vi "Close.vi"(8 "error in (no error)":errorcluster, 11 "Digital Output in":refnum<class "Digital Output.lvclass">) -> (0 "error out":errorcluster)   [LabVIEW 2021, in "Digital Output.lvlib" / "Digital Output.lvclass"]
uses:
  Digital Output.lvclass
  Digital Output.lvclass/Digital Output.ctl
  <vilib>/DAQmx/write.llb/DAQmx Write (Digital Bool 1Line 1Point).vi
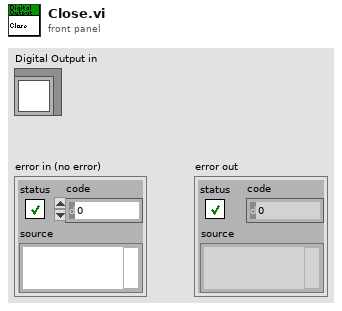
[diagram p1: front panel]
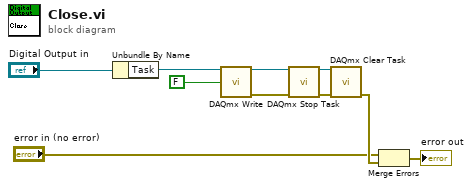
[diagram p0: block diagram]
diagram:
  n1 = Unbundle By Name("Digital Output in") -> ("Task"=w6:refnum<k21>)
  n2 = call-poly <vilib>:"DAQmx Write.vi"("task/channels in"=w6, "data"=FALSE) -> ("task out"=w5:refnum<k21>, "error out"=w7:errorcluster)  [unwired: 11 in, 1 out]
  n3 = call <vilib>:"DAQmx Stop Task.vi"("task/channels in"=w5, "error in"=w7) -> ("task out"=w10:refnum<k21>, "error out"=w9:errorcluster)  [unwired: 12 in]
  n4 = call <vilib>:"DAQmx Clear Task.vi"("task in"=w10, "error in"=w9) -> ("error out"=w8:errorcluster)  [unwired: 13 in]
  n5 = Merge Errors("error in (no error)", w8) -> (→"error out":errorcluster)
